vi "ConnectionData_Write.vi"(1 "ConnectionDataIN":T1={"DeviceIDCtrl"=1, "ProtocolCtrl"=enum."Modbus RTU", "COMportCtrl"="COM2", "IPCtrl"="", "serial master instance"=refnum, "ConnectionStatusIndicator"=FALSE}, 2 "AxisNo":u16) -> ()   [LabVIEW 2020, in "SMCD14_lib.lvlib"]
uses:
  SMCD14_lib.lvlib
  ConnectionData_typedef.ctl
  <vilib>/Modbus/master/Modbus Master.lvclass
  Globals.vi
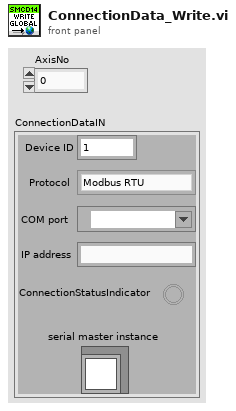
[diagram p1: front panel]
types:
  T1 = typedef "SMCD14_lib.lvlib/ConnectionData_typedef.ctl" = cluster{"DeviceIDCtrl":u16, "ProtocolCtrl":enum16{"Modbus RTU", "Modbus TCP", ""}, "COMportCtrl":refnum<visa-resource-name>, "IPCtrl":string, "serial master instance":refnum<class "Modbus Master.lvclass">, "ConnectionStatusIndicator":bool}
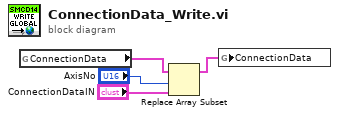
[diagram p0: block diagram]
diagram:
  n1 = global read "Globals.vi" "ConnectionData"() -> (w4:T1[])
  n2 = Replace Array Subset(array=w4, new element="ConnectionDataIN", index="AxisNo") -> (w3:T1[])
  n3 = global write "Globals.vi" "ConnectionData"(w3) -> ()
